vi "sub 1.vi"(8 "error in (no error)":errorcluster, 11 "File Refnum In":refnum<file>) -> (0 "error out":errorcluster)   [LabVIEW 2015]
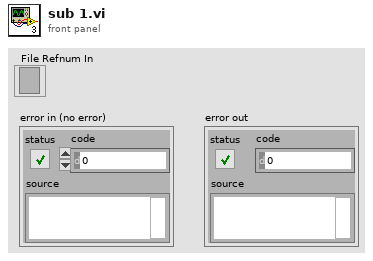
[diagram p1: front panel]
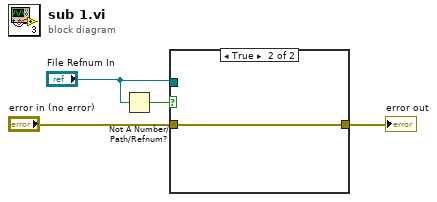
[diagram p0: block diagram]
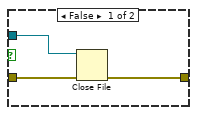
[diagram p2: hidden frame]
diagram:
  n1 = Not A Number/Path/Refnum?(number/path/refnum="File Refnum In") -> (NaN/Path/Refnum?=w3:bool)
  n2 = case shown="True" w3 {
    tunnel: "File Refnum In" -> [w7 _]
    tunnel: "error in (no error)" -> [w6 w8]
    tunnel: [w5 w8] -> w1
    frame False {
      n3 = Close File(refnum=w7, error in=w6) -> (error out=w5:errorcluster)  [unwired: 1 out]
    }
    frame True {
    }
  }
  "error out" <- w1
